vi "_Extract Mass Range Data.vi"(5 "MR# (0)":i32, 6 "Expt# (0)":i32, 7 "Spectrum":dbl[](array[numeric])) -> (3 "MR Data":cluster{dbl[], dbl[]})   [LabVIEW 2012]
uses:
  Configuration/_Global Configuration.vi
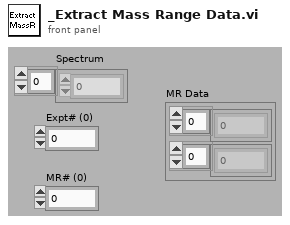
[diagram p1: front panel]
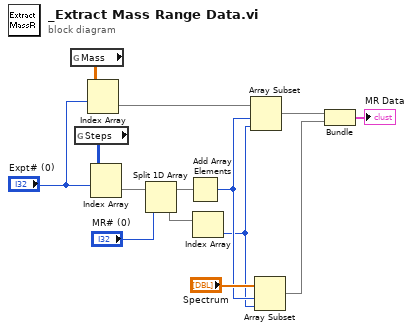
[diagram p0: block diagram]
diagram:
  n1 = global read "_Global Configuration.vi" "Mass"() -> (w9:dbl[][])
  n2 = global read "_Global Configuration.vi" "Steps"() -> (w14:i32[][])
  n3 = Index Array(array=w9, index (row)="Expt# (0)") -> (element=w7:dbl[])  [unwired: 1 in]
  n4 = Index Array(array=w14, index (row)="Expt# (0)") -> (element=w13:i32[])  [unwired: 1 in]
  n5 = Split 1D Array(array=w13, index="MR# (0)") -> (first subarray=w11:i32[], second subarray=w10:i32[])
  n6 = Add Array Elements(numeric array=w11) -> (sum=w5:i32)
  n7 = Index Array(array=w10) -> (element=w4:i32)  [unwired: 1 in]
  n8 = Array Subset(array=w7, index=w5, length=w4) -> (w3:dbl[])
  n9 = Array Subset(array="Spectrum", index=w5, length=w4) -> (w2:dbl[])
  n10 = Bundle(w3, w2) -> (→"MR Data":cluster{dbl[], dbl[]})  [unwired: 1 out]
